vi "Write Offset Values to Default.vi"(6 "error in":errorcluster, 8 "MaxRead":i32, 9 "Channel in":u16) -> (0 "error out":errorcluster, 1 "Messages":T1(array[cluster]), 2 "Pass":bool, 3 "Channel out":u16)   [LabVIEW 2023]
uses:
  4f930f32-d09a-43ef-bca1-8b214b378bd5.vi
  e8470de1-fa2d-4ee3-b50e-96bd89dc731f.vi
  Communication/PCAN2023/PCAN API.lvlib
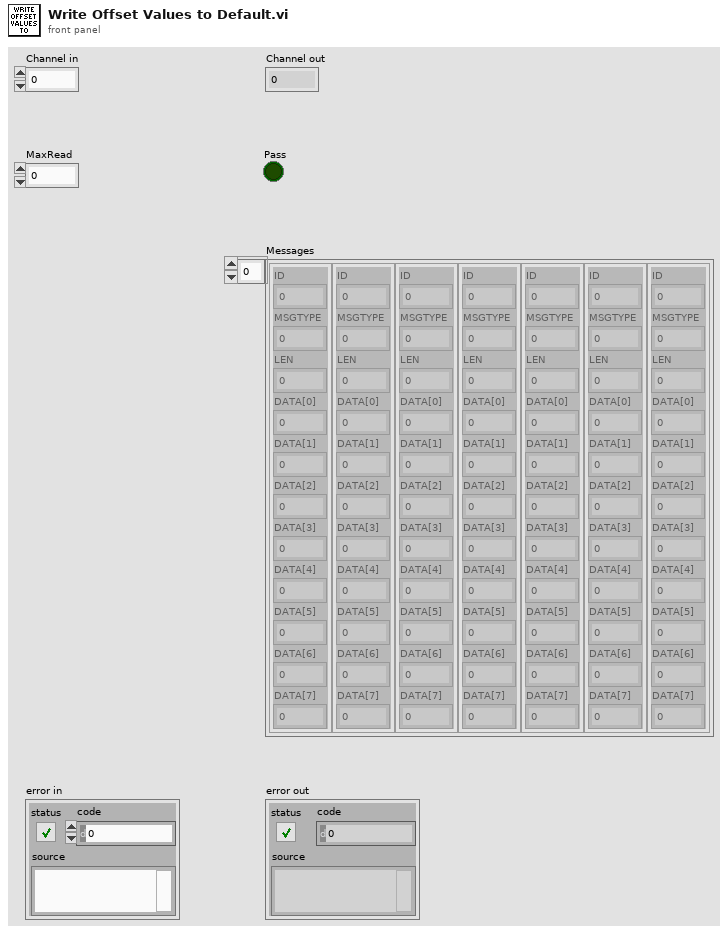
[diagram p1: front panel]
types:
  T1 = cluster{"ID":u32, "MSGTYPE":u8, "LEN":u8, "DATA[0]":u8, "DATA[1]":u8, "DATA[2]":u8, "DATA[3]":u8, "DATA[4]":u8, "DATA[5]":u8, "DATA[6]":u8, "DATA[7]":u8}[]
  T2 = cluster{"ID":u32, "MSGTYPE":u8, "LEN":u8, "DATA[0]":u8, "DATA[1]":u8, "DATA[2]":u8, "DATA[3]":u8, "DATA[4]":u8, "DATA[5]":u8, "DATA[6]":u8, "DATA[7]":u8}
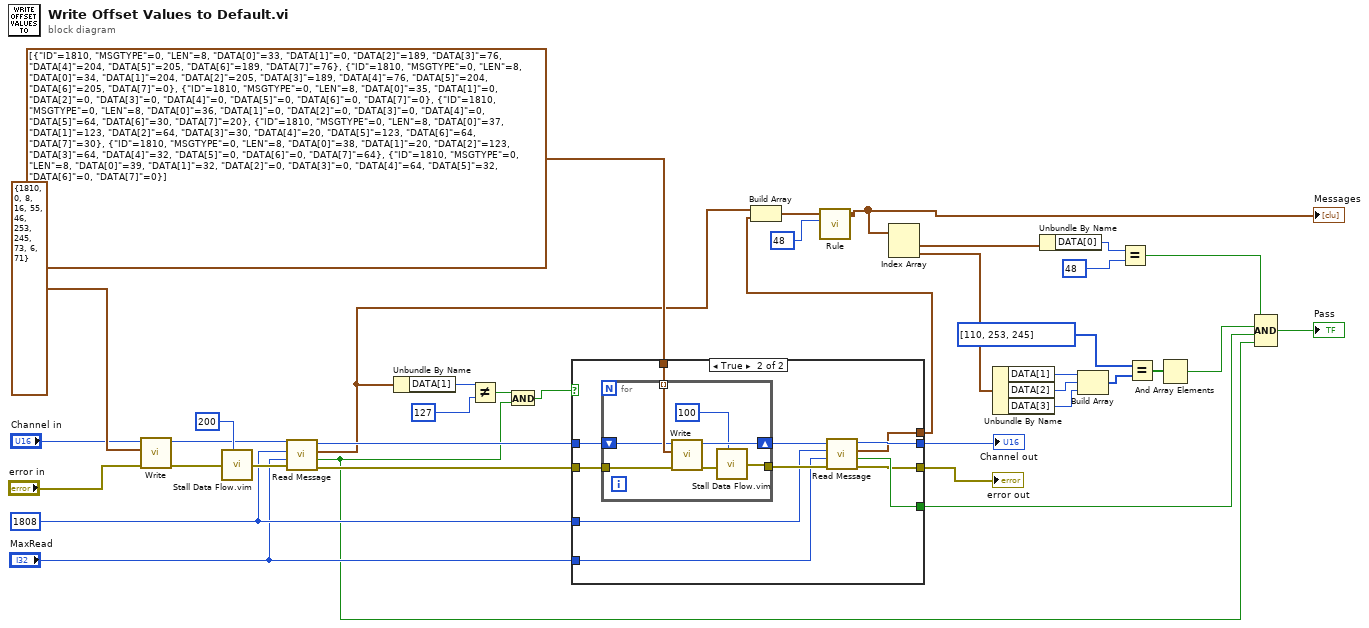
[diagram p0: block diagram]
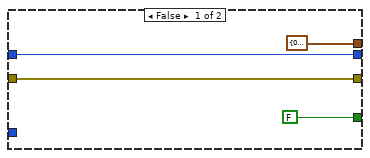
[diagram p2: hidden frame]
diagram:
  (unwired) u32 200 ("milliseconds to wait")
  w10 = u32 1808 ("ID")
  n1 = call "Write.vi"("error in"="error in", "MessageBuffer"=T2 {"ID"=1810, "MSGTYPE"=0, "LEN"=8, "DATA[0]"=16, "DATA[1]"=55, "DATA[2]"=46, "DATA[3]"=253, "DATA[4]"=245, "DATA[5]"=73, "DATA[6]"=6, "DATA[7]"=71}, "Channel"="Channel in") -> ("error out"=w25:errorcluster, "Channel out"=w15:u16)  [unwired: 5 in, 2 out]
  n2 = call "Stall Data Flow.vim"("value in"=w25, "milliseconds to wait"=u32 200) -> ("value out"=w13:errorcluster)  [unwired: 1 out]
  n3 = call "Read Message.vi"("error in"=w13, "MaxRead"="MaxRead", "ID"=w10, "Channel in"=w15) -> ("error out"=w12:errorcluster, "Passed"=w6:bool, "Last Message"=w11:T2, "Channel out"=w14:u16)  [unwired: 3 in, 1 out]
  n4 = Unbundle By Name(w11) -> ("DATA[1]"=w16:u8)
  n5 = Not Equal?(x=w16, y=u8 127) -> (x != y?=w8:bool)
  n6 = And(x=w8, y=w6) -> (x .and. y?=w7:bool)
  n7 = case shown="True" w7 {
    tunnel: T1 [{"ID"=1810, "MSGTYPE"=0, "LEN"=8, "DATA[0]"=33, "DATA[1]"=0, "DATA[2]"=189, "DATA[3]"=76, "DATA[4]"=204, "DATA[5]"=205, "DATA[6]"=189, "DATA[7]"=76}, {"ID"=1810, "MSGTYPE"=0, "LEN"=8, "DATA[0]"=34, "DATA[1]"=204, "DATA[2]"=205, "DATA[3]"=189, "DATA[4]"=76, "DATA[5]"=204, "DATA[6]"=205, "DATA[7]"=0}, {"ID"=1810, "MSGTYPE"=0, "LEN"=8, "DATA[0]"=35, "DATA[1]"=0, "DATA[2]"=0, "DATA[3]"=0, "DATA[4]"=0, "DATA[5]"=0, "DATA[6]"=0, "DATA[7]"=0}, {"ID"=1810, "MSGTYPE"=0, "LEN"=8, "DATA[0]"=36, "DATA[1]"=0, "DATA[2]"=0, "DATA[3]"=0, "DATA[4]"=0, "DATA[5]"=64, "DATA[6]"=30, "DATA[7]"=20}, {"ID"=1810, "MSGTYPE"=0, "LEN"=8, "DATA[0]"=37, "DATA[1]"=123, "DATA[2]"=64, "DATA[3]"=30, "DATA[4]"=20, "DATA[5]"=123, "DATA[6]"=64, "DATA[7]"=30}, {"ID"=1810, "MSGTYPE"=0, "LEN"=8, "DATA[0]"=38, "DATA[1]"=20, "DATA[2]"=123, "DATA[3]"=64, "DATA[4]"=32, "DATA[5]"=0, "DATA[6]"=0, "DATA[7]"=64}, {"ID"=1810, "MSGTYPE"=0, "LEN"=8, "DATA[0]"=39, "DATA[1]"=32, "DATA[2]"=0, "DATA[3]"=0, "DATA[4]"=64, "DATA[5]"=32, "DATA[6]"=0, "DATA[7]"=0}] ("MessageBuffer") -> [_ w53]
    tunnel: w14 -> [w41 w52]
    tunnel: w12 -> [w40 w51]
    tunnel: [w40 w46] -> w21
    tunnel: [FALSE w47] -> w20
    tunnel: [w41 w49] -> w19
    tunnel: [T2 {"ID"=0, "MSGTYPE"=0, "LEN"=0, "DATA[0]"=0, "DATA[1]"=0, "DATA[2]"=0, "DATA[3]"=0, "DATA[4]"=0, "DATA[5]"=0, "DATA[6]"=0, "DATA[7]"=0} ("MessageBuffer out") w48] -> w18
    tunnel: w10 -> [_ w44]
    tunnel: "MaxRead" -> [_ w43]
    frame False {
    }
    frame True {
      n8 = for {
        tunnel: w53 -> [w60] mode=indexing
        shift-right: [w57] -> w50
        shift-left: w52 -> [w59]
        tunnel: w51 -> [w58]
        tunnel: [w54] -> w45
        n9 = call "Write.vi"("error in"=w58, "MessageBuffer"=w60, "Channel"=w59) -> ("error out"=w55:errorcluster, "Channel out"=w57:u16)  [unwired: 5 in, 2 out]
        n10 = call "Stall Data Flow.vim"("value in"=w55, "milliseconds to wait"=u32 100) -> ("value out"=w54:errorcluster)  [unwired: 1 out]
      }
      n11 = call "Read Message.vi"("error in"=w45, "MaxRead"=w43, "ID"=w44, "Channel in"=w50) -> ("error out"=w46:errorcluster, "Passed"=w47:bool, "Last Message"=w48:T2, "Channel out"=w49:u16)  [unwired: 3 in, 1 out]
    }
  }
  "error out" <- w21
  "Channel out" <- w19
  n12 = Build Array(w11, w18) -> (w5:T1)
  n13 = call "Rule.vi"("Case"=u8 48 ("y"), "Array in"=w5) -> ("Array out"=w3:T1)  [unwired: 9 in]
  "Messages" <- w3
  n14 = Index Array(array=w3) -> (element #1=w2:T2, element #2=w1:T2)  [unwired: 2 in]
  n15 = Unbundle By Name(w1) -> ("DATA[1]"=w32:u8, "DATA[2]"=w31:u8, "DATA[3]"=w30:u8)
  n16 = Unbundle By Name(w2) -> ("DATA[0]"=w24:u8)
  n17 = Build Array(w32, w31, w30) -> (w29:u8[])
  n18 = Equal?(x=w24, y=u8 48) -> (x = y?=w22:bool)
  n19 = Equal?(x=u8[] [110, 253, 245], y=w29) -> (x = y?=w34:bool[])
  n20 = And Array Elements(Boolean array=w34) -> (logical AND=w28:bool)
  n21 = Compound Arithmetic op=AND(w22, w28, w20, w6) -> (→"Pass":bool)
